vi "Create log msg from generic msg.vi"(10 "Thread":T1, 11 "variant":variant) -> ()   [LabVIEW 2015]
uses:
  Controls/Log Thread Name.ctl
  Controls/Generic Log Massage.ctl
  LP Globals.vi
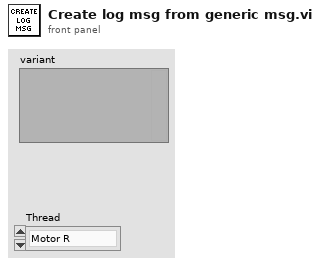
[diagram p1: front panel]
types:
  T1 = typedef "Log Thread Name.ctl" = enum16{"Motor R", "Generic", "Motor P", "Motor Y", "StreamClient", "Stream Server", "Sequencer"}
  T2 = typedef "Generic Log Massage.ctl" = cluster{"Thread":T1, "Msg":string}
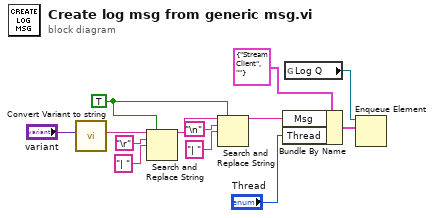
[diagram p0: block diagram]
diagram:
  w6 = TRUE ("replace all? (F)")
  n1 = call "Convert Variant to string.vi"("variant"="variant") -> ("data string"=w1:string)  [unwired: 10 in]
  n2 = Search and Replace String(replace all?=w6, input string=w1, search string="\r", replace string="| " ("replace string (\"\")")) -> (result string=w7:string)  [unwired: 4 in, 3 out]
  n3 = Search and Replace String(replace all?=w6, input string=w7, search string="\n", replace string="| " ("replace string (\"\")")) -> (result string=w3:string)  [unwired: 4 in, 3 out]
  n4 = Bundle By Name(cluster=T2 {"Thread"=enum."StreamClient", "Msg"=""} ("element"), "Msg"=w3, "Thread"="Thread") -> (w13:T2)
  n5 = global read "LP Globals.vi" "Log Q"() -> (w11:refnum<queue>)
  n6 = Enqueue Element(queue=w11, element=w13) -> ()  [unwired: 2 in, 3 out]
